vi "GEOM_GetIniConstants.vi"(8 "error in (no error)":errorcluster, 10 "fpa  file":path=path "/home/ArcVIEW/Modules/GEOM/public/database") -> (0 "error out":errorcluster)   [LabVIEW 2016]
uses:
  GEOM_VAR_action.ctl
  <vilib>/Utility/config.llb/Read Key (String).vi
  <vilib>/Utility/config.llb/NI_LVConfig.lvlib
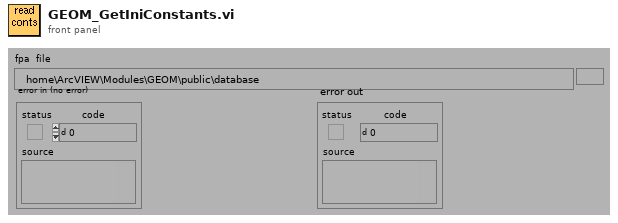
[diagram p1: front panel]
types:
  T1 = typedef "GEOM_VAR_action.ctl" = enum16{"read", "write"}
  T2 = typedef "NI_LVConfig.lvlib/Config Data RefNum.ctl" = refnum<k1>
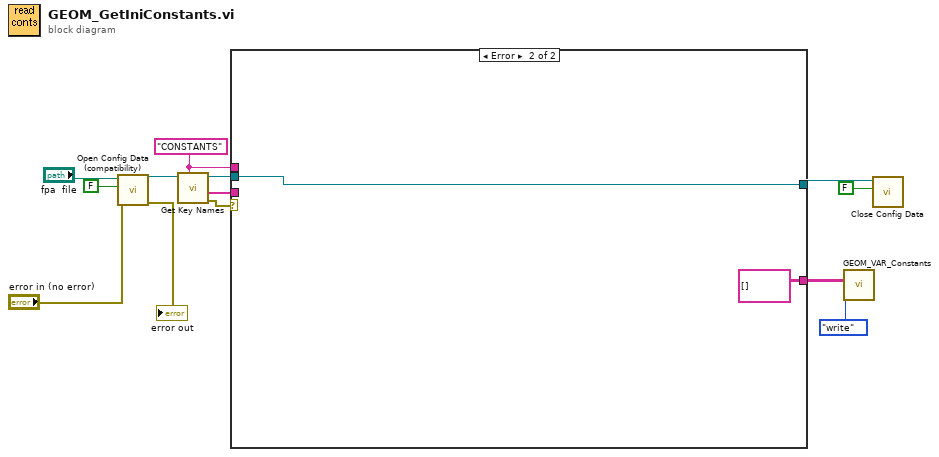
[diagram p0: block diagram]
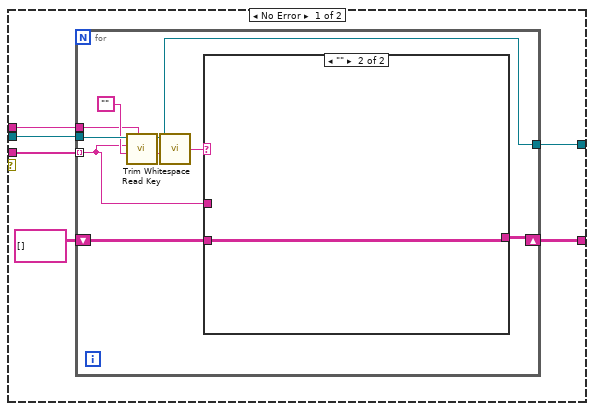
[diagram p2: hidden frame]
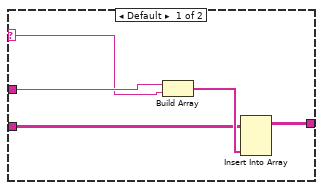
[diagram p3: hidden frame]
diagram:
  w5 = "CONSTANTS" ("section")
  n1 = call <vilib>:"Open Config Data (compatibility).vi"("error in (no error)"="error in (no error)", "create file if necessary (T)"=FALSE ("create file if necessary? (T)"), "configuration file path"="fpa  file") -> ("error out"=→"error out":errorcluster, "refnum"=w11:T2)  [unwired: 6 in, 1 out]
  n2 = call <vilib>:"Get Key Names.vi"("section"=w5, "refnum"=w11) -> ("error out"=w10:errorcluster, "key names"=w6:string[], "refnum out"=w9:T2)  [unwired: 1 in, 6 out]
  n3 = case shown="Error" w10 {
    tunnel: w9 -> [w19 w36]
    tunnel: [w14 w36] -> w8
    tunnel: w6 -> [w18 _]
    tunnel: w5 -> [w17 _]
    tunnel: [w15 string[][] []] -> w4
    frame No Error {
      n4 = for {
        tunnel: w19 -> [w28]
        tunnel: w18 -> [w23] mode=indexing
        shift-right: [w22] -> w15
        shift-left: string[][] [] -> [w21]
        tunnel: w17 -> [w24]
        tunnel: [w20] -> w14
        n5 = call-poly <vilib>:"Read Key.vi"("section"=w24, "default value"="", "key"=w23, "refnum"=w28) -> ("value"=w26:string, "refnum out"=w20:T2)  [unwired: 2 in, 4 out]
        n6 = call <vilib>:"Trim Whitespace.vi"("string"=w26) -> ("trimmed string"=w25:string)  [unwired: 1 in]
        n7 = case shown="\"\"" w25 {
          selector: w25 -> [w32 _]
          tunnel: w23 -> [w33 _]
          tunnel: [w30 w34] -> w22
          tunnel: w21 -> [w29 w34]
          frame Default {
            n8 = Build Array(w33, w32) -> (w31:string[])
            n9 = Insert Into Array(array=w29, new element=w31) -> (w30:string[][])  [unwired: 2 in]
          }
          frame "" {
          }
        }
      }
    }
    frame Error {
    }
  }
  n10 = call "GEOM_VAR_Constants.vi"("Action"=GEOM_VAR_action."write", "GEOM_constants"=w4) -> ()  [unwired: 10 out]
  n11 = call <vilib>:"Close Config Data.vi"("write file if changed (T)"=FALSE ("write configuration file? (T)"), "refnum"=w8) -> ()  [unwired: 1 in, 9 out]
